vi "ReviewQnsPaper2(SubVI).vi"(11 "connection reference":T2) -> (0 "close?":bool, 3 "connection reference out":T2)   [LabVIEW 2013]
uses:
  <vilib>/addons/database/Connection.llb/Conn ObjectReference.ctl
  <vilib>/Utility/miscctls.llb/LVBoundsTypeDef.ctl
  Dropbox/Programs/FYP_LabviewGlobal(SubVI).vi
  <vilib>/addons/database/NI_Database_API.lvlib
panel:
  out "Image_RandomisedMCQ_Options":picture
  in  "SelectQn":T1(radio)
  in  "Close":bool
  out "Marks%":dbl
  out "TotalMarks":string
  # "% )"
  # "Your Score is :"
  # "("
  # "Questions:"
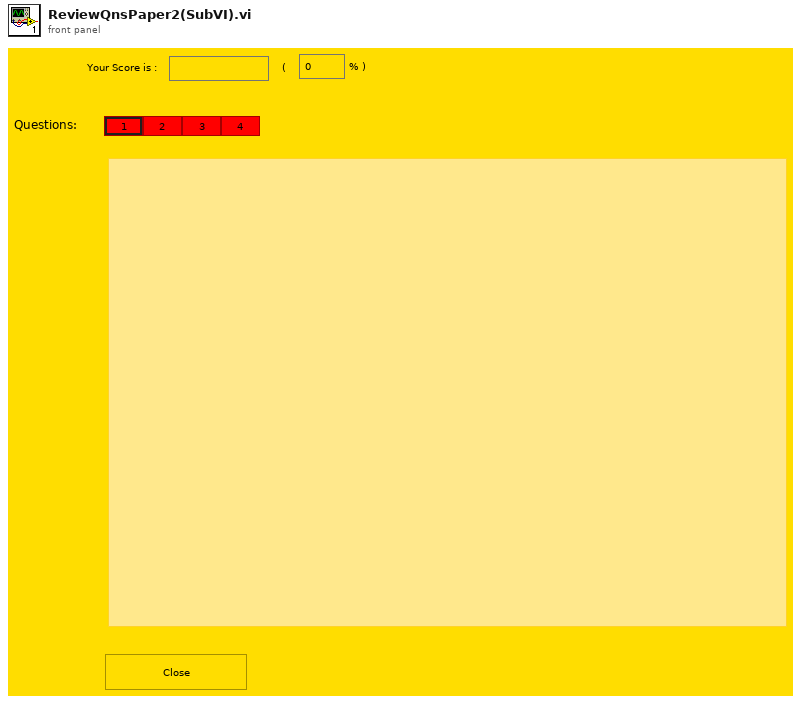
[diagram p1: front panel]
types:
  T1 = enum32{"1", "2", "3", "4", "5", "6", "7", "8", "9", "10", "11", "12", "13", "14", "15", "16", "17", "18", "19", "20"}
  T2 = typedef "NI_Database_API.lvlib/Conn ObjectReference.ctl" = refnum<k1>
  T3 = typedef "LVBoundsTypeDef.ctl" = cluster{"Width":u32, "Height":u32}
  T4 = typedef "imagedata.ctl" = cluster{"image type":i32, "image depth":i32, "image":u8[], "mask":u8[], "colors":u32[], "Rectangle":cluster{"left":i16, "top":i16, "right":i16, "bottom":i16}}
  T5 = typedef "LVPositionTypeDef.ctl" = cluster{"Left":i32, "Top":i32}
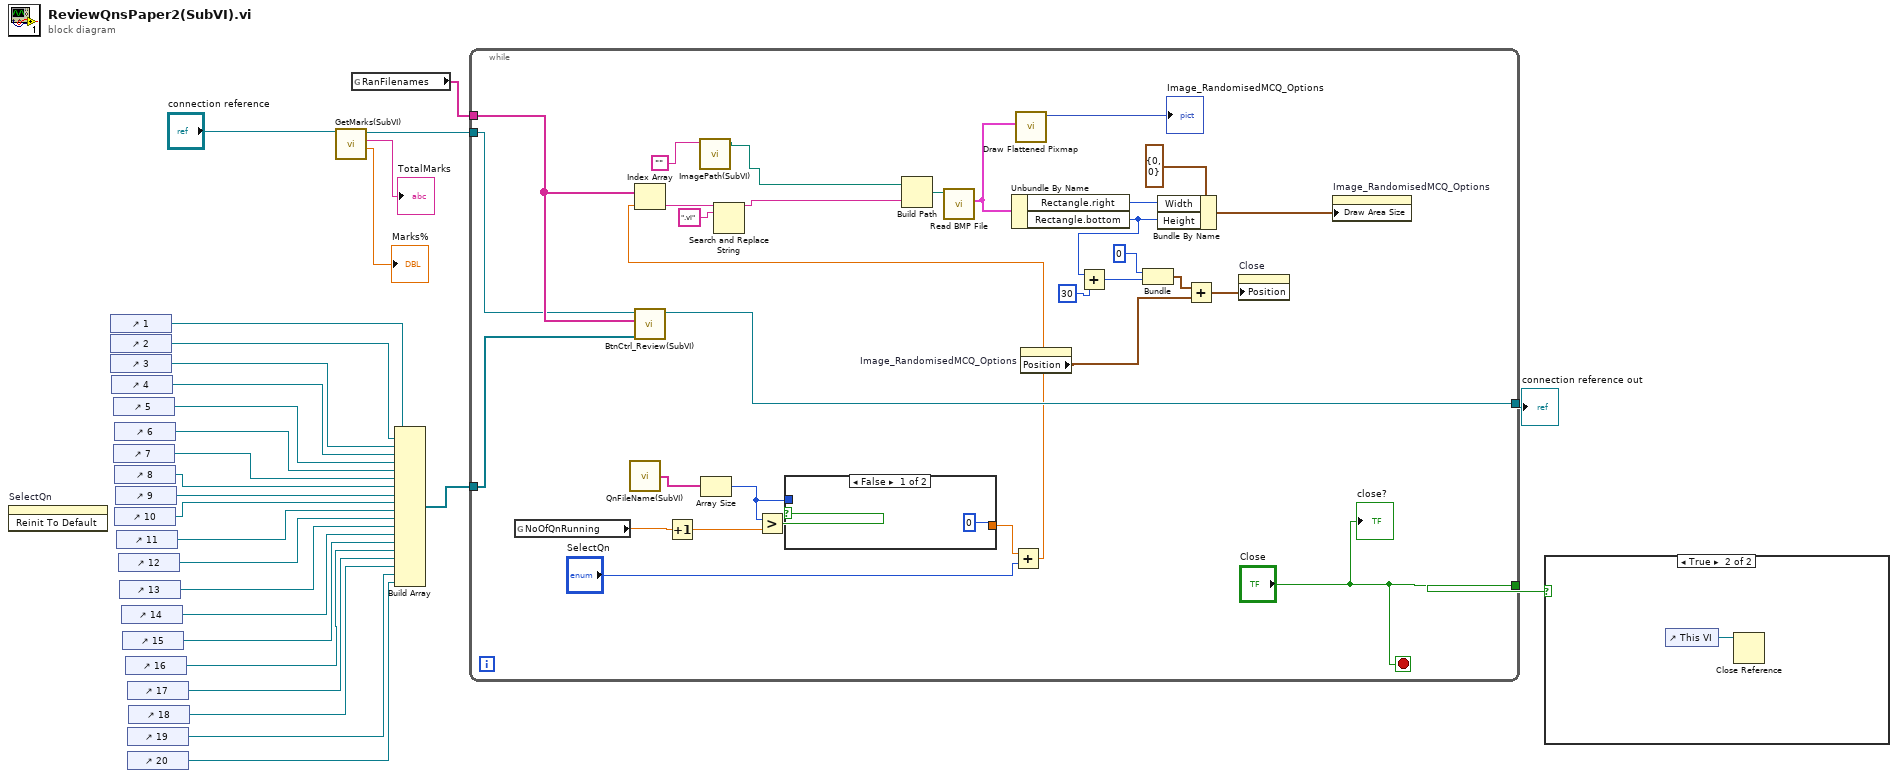
[diagram p0: block diagram]
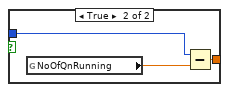
[diagram p3: hidden frame]
diagram:
  n1 = invoke on="SelectQn" class="RadioBtnsControl (strict)" method="Reinit To Default"() -> ()  [unwired: 3 in, 3 out]
  n2 = control-ref of="1"() -> (w20:refnum<vi>)
  n3 = control-ref of="2"() -> (w19:refnum<vi>)
  n4 = control-ref of="3"() -> (w18:refnum<vi>)
  n5 = control-ref of="4"() -> (w17:refnum<vi>)
  n6 = control-ref of="5"() -> (w16:refnum<vi>)
  n7 = control-ref of="7"() -> (w14:refnum<vi>)
  n8 = control-ref of="6"() -> (w15:refnum<vi>)
  n9 = control-ref of="8"() -> (w13:refnum<vi>)
  n10 = control-ref of="10"() -> (w11:refnum<vi>)
  n11 = control-ref of="9"() -> (w12:refnum<vi>)
  n12 = control-ref of="11"() -> (w10:refnum<vi>)
  n13 = control-ref of="12"() -> (w9:refnum<vi>)
  n14 = control-ref of="13"() -> (w8:refnum<vi>)
  n15 = control-ref of="14"() -> (w7:refnum<vi>)
  n16 = control-ref of="15"() -> (w6:refnum<vi>)
  n17 = control-ref of="16"() -> (w1:refnum<vi>)
  n18 = control-ref of="17"() -> (w2:refnum<vi>)
  n19 = control-ref of="19"() -> (w4:refnum<vi>)
  n20 = control-ref of="20"() -> (w5:refnum<vi>)
  n21 = control-ref of="18"() -> (w3:refnum<vi>)
  n22 = call "GetMarks(SubVI).vi"("connection reference 3"="connection reference") -> ("Marks%"=→"Marks%":dbl, "TotalMarks"=→"TotalMarks":string, "connection reference 2"=w24:T2)  [unwired: 8 in]
  n23 = global read "FYP_LabviewGlobal(SubVI).vi" "RanFilenames"() -> (w25:string[])
  n24 = Build Array(w20, w19, w18, w17, w16, w15, w14, w13, w12, w11, w10, w9, w8, w7, w6, w1, w2, w3, w4, w5) -> (w23:refnum<vi>[])
  n25 = while {
    tunnel: w25 -> [w43]
    tunnel: w24 -> [w32]
    tunnel: w23 -> [w42]
    tunnel: [w41] -> w22
    tunnel: ["Close"] -> w21
    stop <- "Close" stop-if-true
    n26 = global read "FYP_LabviewGlobal(SubVI).vi" "NoOfQnRunning"() -> (w40:dbl)
    n27 = call "QnFileName(SubVI).vi"() -> ("FileNames"=w59:string[])
    n28 = call "BtnCtrl_Review(SubVI).vi"("ButtonControlArray"=w42, "RanFilenames"=w43, "connection reference"=w32) -> ("connection reference out"=w41:T2)  [unwired: 8 in]
    n29 = Increment(x=w40) -> (x+1=w39:dbl)
    n30 = call "ImagePath(SubVI).vi"("Name"="") -> ("ImagePath"=w29:path)  [unwired: 10 in]
    n31 = Array Size(array=w59) -> (size(s)=w56:i32)
    n32 = Greater?(x=w56, y=w39) -> (0:w58:bool)
    n33 = case shown="False" w58 {
      tunnel: w56 -> [_ w63]
      tunnel: [0 w62] -> w57
      frame False {
      }
      frame True {
        n34 = global read "FYP_LabviewGlobal(SubVI).vi" "NoOfQnRunning"() -> (w61:dbl)
        n35 = Subtract(x=w63, y=w61) -> (x-y=w62:dbl)
      }
    }
    n36 = Add(x=w57, y="SelectQn") -> (x+y=w31:dbl)
    n37 = Index Array(array=w43, index=w31) -> (element=w54:string)
    n38 = Search and Replace String(input string=w54, search string=".vi" ("substring (\"\")")) -> (result string=w52:string)  [unwired: 6 in, 3 out]
    n39 = Build Path(base path=w29, name or relative path=w52) -> (appended path=w53:path)
    n40 = call <vilib>:"Read BMP File.vi"("path to BMP file"=w53) -> ("image data"=w51:T4)  [unwired: 8 in, 2 out]
    n41 = Unbundle By Name(w51) -> ("Rectangle.right"=w45:i16, "Rectangle.bottom"=w35:i16)
    n42 = call <vilib>:"Draw Flattened Pixmap.vi"("image data"=w51) -> ("new picture"=→"Image_RandomisedMCQ_Options":picture)  [unwired: 8 in]
    n43 = property on="Image_RandomisedMCQ_Options" class="Pict"() -> ("Position"=w37:T5)  [unwired: 2 in, 2 out]
    n44 = Add(x=w35, y=30) -> (x+y=w33:i32)
    n45 = Bundle(0, w33) -> (w49:cluster{i32, i32})  [unwired: 1 in]
    n46 = Bundle By Name "Bundle By Name"(cluster=T3 {"Width"=0, "Height"=0} ("Draw Area Size"), "Width"=w45, "Height"=w35) -> (w36:T3)
    n47 = Add(x=w49, y=w37) -> (x+y=w48:T5)
    n48 = property on="Close" class="Bool"("Position"=w48) -> ()  [unwired: 2 in, 2 out]
    n49 = property on="Image_RandomisedMCQ_Options" class="Pict"("Draw Area Size"=w36) -> ()  [unwired: 2 in, 2 out]
    "close?" <- "Close"
  }
  "connection reference out" <- w22
  n50 = case shown="True" w21 {
    frame False {
    }
    frame True {
      n51 = control-ref of="This VI"() -> (w64:refnum<vi>)
      n52 = Close Reference(reference=w64) -> ()  [unwired: 1 in, 1 out]
    }
  }
